vi "update.vi"(8 "error in":errorcluster, 10 "settings cluster":T2, 11 "FPGA VI ref":T1) -> (0 "error out":errorcluster)   [LabVIEW 2010]
uses:
  type definitions/settings_cluster.ctl
  common_typedefs/channels_cluster.ctl
  type definitions/gate_cluster.ctl
  common_typedefs/gate_parameters_cluster.ctl
  FPGA_VI_reference.ctl
  <vilib>/rvi/interface/nirviReadWriteControl/nirviReadWriteControl.xnode
  <vilib>/rvi/interface/common/niFpgaNodeNameForErrorReporting.ctl
  <vilib>/rvi/errors/niLvFpgaWhatHappensToTopLevelVI.ctl
  <vilib>/Utility/error.llb/Error Cluster From Error Code.vi
  <vilib>/rvi/errors/niLvFpgaAdjustHostInterfaceError.vi
  NiFpgaLv.dll
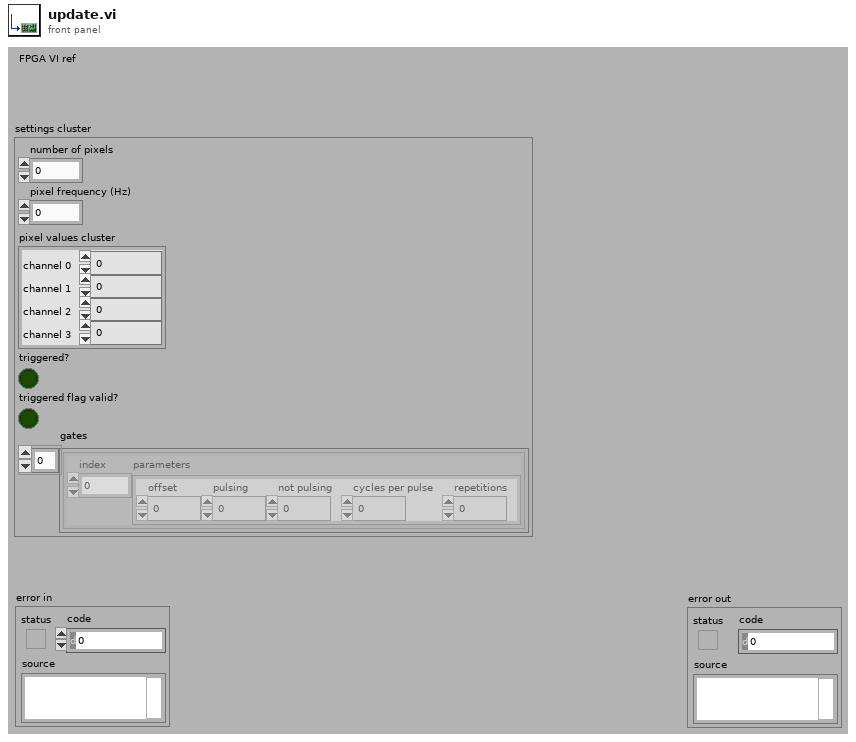
[diagram p1: front panel]
types:
  T1 = typedef "FPGA_VI_reference.ctl" = refnum<k20>
  T2 = typedef "settings_cluster.ctl" = cluster{"number of pixels":i64, "pixel frequency (Hz)":dbl, "pixel values cluster":T3, "triggered?":bool, "triggered flag valid?":bool, "gates":T4[]}
  T3 = typedef "channels_cluster.ctl" = cluster{"channel 0":u32, "channel 1":u32, "channel 2":u32, "channel 3":u32}
  T4 = typedef "gate_cluster.ctl" = cluster{"index":i32, "parameters":T5}
  T5 = typedef "gate_parameters_cluster.ctl" = cluster{"offset":i64, "pulsing":i64, "not pulsing":i64, "cycles per pulse":i64, "repetitions":i64}
  T6 = typedef "niFpgaNodeNameForErrorReporting.ctl" = enum16{"Open FPGA VI Reference", "Read/Write Control", "Invoke Method: Abort", "Invoke Method: Acknowledge IRQ", "Invoke Method: Download", "Invoke Method: FIFO.Configure", "Invoke Method: FIFO.Read", "Invoke Method: FIFO.Start", "Invoke Method: FIFO.Stop", "Invoke Method: FIFO.Write", "Invoke Method: Reset", "Invoke Method: Run", "Invoke Method: Wait on IRQ", "Close FPGA VI Reference"}
  T7 = typedef "niLvFpgaWhatHappensToTopLevelVI.ctl" = enum16{"top level VI scripted behind XNode", "top level VI inlined behind XNode"}
  T8 = cluster{"channel 0":u32, "channel 1":u32, "channel 2":u32, "channel 3":u32}
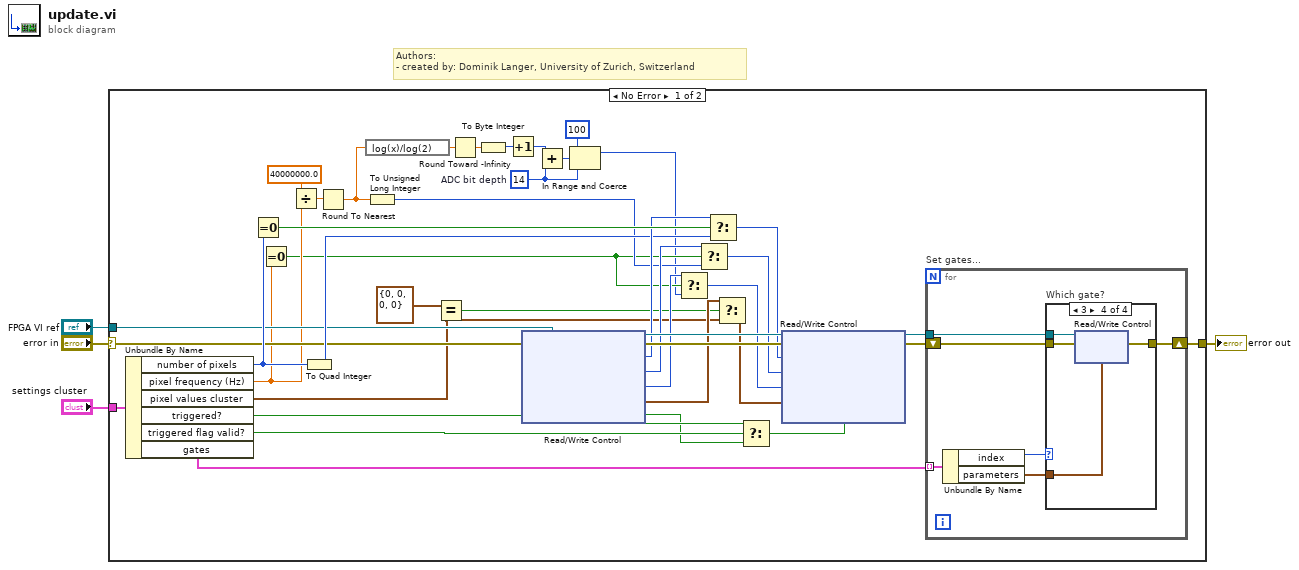
[diagram p0: block diagram]
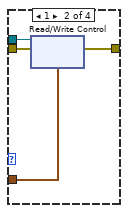
[diagram p3: hidden frame]
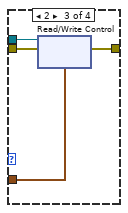
[diagram p4: hidden frame]
diagram:
  # "Authors: \n- created by: Dominik Langer, University of Zurich, Switzerland"
  n1 = case shown="No Error" "error in" {
    selector: "error in" -> [w30 w486]
    tunnel: "settings cluster" -> [w31 _]
    tunnel: [w20 w486] -> w2
    tunnel: "FPGA VI ref" -> [w29 _]
    frame No Error {
      w11 = i8 14  # ADC bit depth
      n2 = Unbundle By Name(w31) -> ("number of pixels"=w43:i64, "pixel frequency (Hz)"=w17:dbl, "pixel values cluster"=w25:T3, "triggered?"=w33:bool, "triggered flag valid?"=w34:bool, "gates"=w22:T4[])
      n3 = Equal To 0?(x=w43) -> (x = 0?=w42:bool)
      n4 = Equal To 0?(x=w17) -> (x = 0?=w14:bool)
      n5 = Divide(x=40000000.0, y=w17) -> (x/y=w16:dbl)
      n6 = To Quad Integer(1:w43) -> (0:w40:i64)
      n7 = Round To Nearest(number=w16) -> (nearest integer value=w6:dbl)
      n8 = expression code="log(x)/log(2)"(w6) -> (w7:dbl)
      n9 = To Unsigned Long Integer(number=w6) -> (unsigned 32bit integer=w15:u32)
      n10 = Equal?(x=T3 {"channel 0"=0, "channel 1"=0, "channel 2"=0, "channel 3"=0} ("pixel values cluster"), y=w25) -> (x = y?=w23:bool)
      n11 = Round Toward -Infinity(1:w7) -> (0:w8:dbl)
      n12 = To Byte Integer(number=w8) -> (8bit integer=w9:i8)
      n13 = Increment(x=w9) -> (x+1=w10:i8)
      n14 = xnode "Read/Write Control"("FPGA VI Reference In"=w29, "error in"=w30) -> ("FPGA VI Reference Out"=w45:T1, "error out"=w44:errorcluster, "number of pixels"=w41:i64, "iterations per pixel"=w38:u32, "maximum bit depth"=w36:i8, "channel offsets"=w27:T8, "wait for trigger?"=w28:bool)
      n15 = Add(x=w10, y=w11) -> (x+y=w12:i8)
      n16 = In Range and Coerce(upper limit=i8 100, x=w12, lower limit=w11) -> (coerced(x)=w5:i8)  [unwired: 1 out]
      n17 = Select(t=w36, s=w14, f=w5) -> (s? t:f=w35:i8)
      n18 = Select(t=w38, s=w14, f=w15) -> (s? t:f=w37:u32)
      n19 = Select(t=w41, s=w42, f=w40) -> (s? t:f=w39:i64)
      n20 = Select(t=w27, s=w23, f=w25) -> (s? t:f=w26:T3)
      n21 = Select(t=w33, s=w34, f=w28) -> (s? t:f=w32:bool)
      n22 = xnode "Read/Write Control"("FPGA VI Reference In"=w45, "error in"=w44, "number of pixels"=w39, "iterations per pixel"=w37, "maximum bit depth"=w35, "channel offsets"=w26, "wait for trigger?"=w32) -> ("FPGA VI Reference Out"=w19:T1, "error out"=w21:errorcluster)
      n23 = for "Set gates..." {
        tunnel: w22 -> [w51] mode=indexing
        shift-right: [w47] -> w20
        shift-left: w21 -> [w50]
        tunnel: w19 -> [w49]
        n24 = Unbundle By Name(w51) -> ("index"=w48:i32, "parameters"=w46:T5)
        n25 = case "Which gate?" shown="3" w48 {
          tunnel: w50 -> [w52 w56 w102 w150]
          tunnel: w49 -> [_ w55 w104 w151]
          tunnel: [w52 w54 w101 w149] -> w47
          tunnel: w46 -> [_ w53 w103 w152]
          frame Default {
          }
          frame 1 {
            n26 = xnode "Read/Write Control"("FPGA VI Reference In"=w55, "error in"=w56, "gate 1"=w53) -> ("error out"=w54:errorcluster)  [unwired: 1 out]
          }
          frame 2 {
            n27 = xnode "Read/Write Control"("FPGA VI Reference In"=w104, "error in"=w102, "gate 2"=w103) -> ("error out"=w101:errorcluster)  [unwired: 1 out]
          }
          frame 3 {
            n28 = xnode "Read/Write Control"("FPGA VI Reference In"=w151, "error in"=w150, "gate 3"=w152) -> ("error out"=w149:errorcluster)  [unwired: 1 out]
          }
        }
      }
    }
    frame Error {
    }
  }
  "error out" <- w2
